vi "Configure Clock Source.vi"(8 "error in (no error)":errorcluster, 10 "Source (0: Internal)":u16(ring) items=["Internal", "External"], 11 "VISA resource name":refnum<visa-resource-name>) -> (0 "error out":errorcluster, 3 "VISA resource name out":refnum<visa-resource-name>)   [LabVIEW 2015, in "SDG X Series.lvlib"]
doc: "Selects the reference clock source/oscillator for signal generation."
uses:
  <instrlib>/SDG X Series/SDG X Series.lvlib
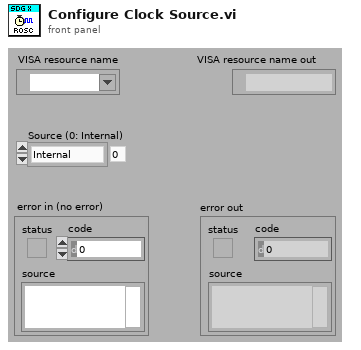
[diagram p1: front panel]
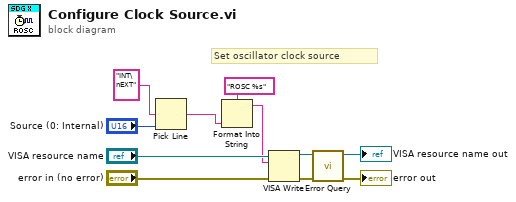
[diagram p0: block diagram]
diagram:
  # "Set oscillator clock source"
  n1 = Pick Line(multi-line string="INT\nEXT", line index="Source (0: Internal)") -> (output string=w6:string)  [unwired: 1 in]
  n2 = Format Into String(format string="ROSC %s", w6) -> (resulting string=w7:string)  [unwired: 2 in, 1 out]
  n3 = VISA Write(VISA resource name="VISA resource name", write buffer=w7, error in (no error)="error in (no error)") -> (VISA resource name out=w3:refnum<visa-resource-name>, error out=w4:errorcluster)  [unwired: 1 out]
  n4 = call <instrlib>:"Error Query.vi"("error in (no error)"=w4, "VISA resource name"=w3) -> ("error out"=→"error out":errorcluster, "VISA resource name out"=→"VISA resource name out":refnum<visa-resource-name>)  [unwired: 6 in, 2 out]
